vi "General - Split Into Lines.vi"(3 "Line Termination Character":string="\r", 4 "String":string) -> (1 "Array":string[](array[string]))   [LabVIEW 2020]
doc: "Splits a string into an array using a defined line termination character."
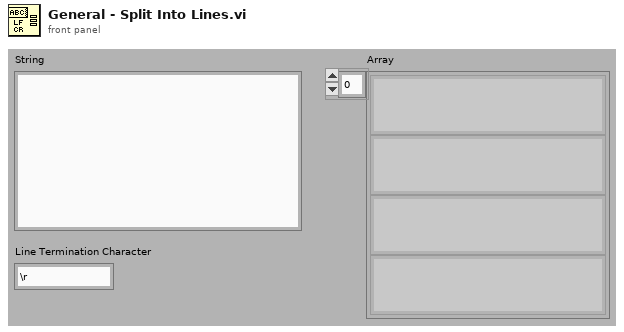
[diagram p1: front panel]
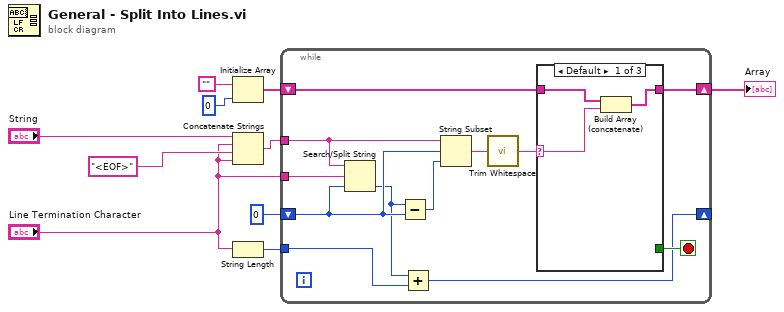
[diagram p0: block diagram]
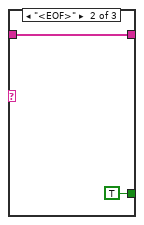
[diagram p2: hidden frame]
diagram:
  n1 = Initialize Array("", 0 ("dimension size")) -> (w5:string[])
  n2 = Concatenate Strings("String", "Line Termination Character", "<EOF>", "Line Termination Character") -> (w10:string)
  n3 = String Length(string="Line Termination Character") -> (length=w1:i32)
  n4 = while {
    tunnel: w10 -> [w22]
    shift-right: [w15] -> _
    shift-left: 0 -> [w20]
    shift-right: [w16] -> w6
    shift-left: w5 -> [w17]
    tunnel: "Line Termination Character" -> [w14]
    tunnel: w1 -> [w11]
    stop <- w18 stop-if-true
    n5 = Search/Split String(string=w22, search string/char (-)=w14, offset (0)=w20) -> (offset of match=w12:i32)  [unwired: 2 out]
    n6 = Subtract(x=w12, y=w20) -> (x-y=w21:i32)
    n7 = Add(x=w12, y=w11) -> (x+y=w15:i32)
    n8 = String Subset(string=w22, offset (0)=w20, length (rest)=w21) -> (substring=w19:string)
    n9 = call <vilib>:"Trim Whitespace.vi"("string"=w19) -> ("trimmed string"=w13:string)  [unwired: 1 in]
    n10 = case shown="Default" w13 {
      selector: w13 -> [w24 _ _]
      tunnel: [_ TRUE _] -> w18
      tunnel: w17 -> [w25 w26 w28]
      tunnel: [w23 w26 w28] -> w16
      frame Default {
        n11 = Build Array (concatenate)(w25, w24) -> (w23:string[])
      }
      frame "<EOF>" {
      }
      frame "" {
      }
    }
  }
  "Array" <- w6
